vi "Start Triggers Time.vi"(0 "time.resources":T3, 5 "rx.parameters":T9={"rx.trigger select"=enum."Software", "rx.trigger enable"=FALSE, "rx.trigger sync enable"=FALSE, "rx.stream enable"=[FALSE, FALSE, FALSE, FALSE], "rx.software trigger"=FALSE, "rx.reset"=FALSE, "rx.abort"=FALSE, "rx.samples to acquire"=0, "rx.data sink"=enum."SFP Port 0", "rx.ddc parameters"=[{"output sample rate"=0.0, "delay"=0.0, "frequency shift"=0.0, "impairments"={"inline gain I"=0.0, "inline gain Q"=0.0, "cross gain I"=0.0, "cross gain Q"=0.0, "pre-gain offset I"=0.0, "pre-gain offset Q"=0.0, "post-gain offset I"=0.0, "post-gain offset Q"=0.0}, "phase"=0.0}, {"output sample rate"=0.0, "delay"=0.0, "frequency shift"=0.0, "impairments"={"inline gain I"=0.0, "inline gain Q"=0.0, "cross gain I"=0.0, "cross gain Q"=0.0, "pre-gain offset I"=0.0, "pre-gain offset Q"=0.0, "post-gain offset I"=0.0, "post-gain offset Q"=0.0}, "phase"=0.0}, {"output sample rate"=0.0, "delay"=0.0, "frequency shift"=0.0, "impairments"={"inline gain I"=0.0, "inline gain Q"=0.0, "cross gain I"=0.0, "cross gain Q"=0.0, "pre-gain offset I"=0.0, "pre-gain offset Q"=0.0, "post-gain offset I"=0.0, "post-gain offset Q"=0.0}, "phase"=0.0}, {"output sample rate"=0.0, "delay"=0.0, "frequency shift"=0.0, "impairments"={"inline gain I"=0.0, "inline gain Q"=0.0, "cross gain I"=0.0, "cross gain Q"=0.0, "pre-gain offset I"=0.0, "pre-gain offset Q"=0.0, "post-gain offset I"=0.0, "post-gain offset Q"=0.0}, "phase"=0.0}]} {"rx.ddc parameters"."frequency shift" format="%#.48g"}, 7 "tx.parameters":T4={"tx.trigger select"=enum."Software", "tx.trigger enable"=FALSE, "tx.trigger sync enable"=FALSE, "tx.stream enable"=[FALSE, FALSE], "tx.software trigger"=FALSE, "tx.reset"=FALSE, "tx.abort"=FALSE, "tx.samples to generate"=0, "tx.data source"=enum."SFP Port 0", "tx.duc parameters"=[{"frequency shift"=0.0, "impairments"={"inline gain I"=0.0, "inline gain Q"=0.0, "cross gain I"=0.0, "cross gain Q"=0.0, "pre-gain offset I"=0.0, "pre-gain offset Q"=0.0, "post-gain offset I"=0.0, "post-gain offset Q"=0.0}, "phase"=0.0, "input sample rate"=0.0, "gain"={"gain I"=0.0, "gain Q"=0.0}, "delay"=0.0}, {"frequency shift"=0.0, "impairments"={"inline gain I"=0.0, "inline gain Q"=0.0, "cross gain I"=0.0, "cross gain Q"=0.0, "pre-gain offset I"=0.0, "pre-gain offset Q"=0.0, "post-gain offset I"=0.0, "post-gain offset Q"=0.0}, "phase"=0.0, "input sample rate"=0.0, "gain"={"gain I"=0.0, "gain Q"=0.0}, "delay"=0.0}]} {"tx.duc parameters"."frequency shift" format="%#.48g"}) -> (4 "rx.start trigger":bool, 6 "tx.start trigger":bool)   [LabVIEW 2018]
doc: "Generates start triggers for Rx and Tx. Start triggers are generated based on which trigger type is selected, whether the stream is enabled, whether triggers are enabled, and whether the triggers are to be synchronized across multiple devices.\n\n<B>Input Parameters</B>\n\n<B>enable stream</B> controls the output of a 'start trigger'.\n\n<B>software trigger</B> is a start trigger asserted by software.\n\n<B>enable trigger</B> controls the output of a 'start trigger'.\n\n<B>enable trigger sync</B> to synchronize a 'start trigger' between multiple devices. The master device sends the 'start trigger' to all the slave devices. If enabled, the slave devices ignore the 'trigger select' because the 'start trigger' from the master device is used instead.\n\n<B>trigger select</B> picks which source to use as the 'start trigger'.\n\n<B>Output Parameters</B>\n\n<B>rx.start trigger</B> is the signal to use at the 'start trigger' for the Rx data path.\n\n<B>tx.start trigger</B> is the signal to use at the 'start trigger' for the Tx data path."
uses:
  Rx Parameters.ctl
  Host/SubVIs/Start Trigger.ctl
  DDC Parameters.ctl
  <instrlib>/_niInstr/DSP/v1/Shared/Public/IQ Impairments.ctl
  Tx Parameters.ctl
  DUC Parameters.ctl
  <instrlib>/_niInstr/DSP/v1/Shared/Public/IQ Gain.ctl
  <instrlib>/niUsrpRio/Time/v1/FPGA/Private/Time Resources.ctl
  <instrlib>/niUsrpRio/Time/v1/FPGA/Private/Future Event Resources.ctl
  <instrlib>/_niInstr/DSP/v1/Shared/niInstr DSP v1 Shared.lvlib
  <instrlib>/niUsrpRio/Time/v1/FPGA/niUsrpRio Time v1 FPGA.lvlib
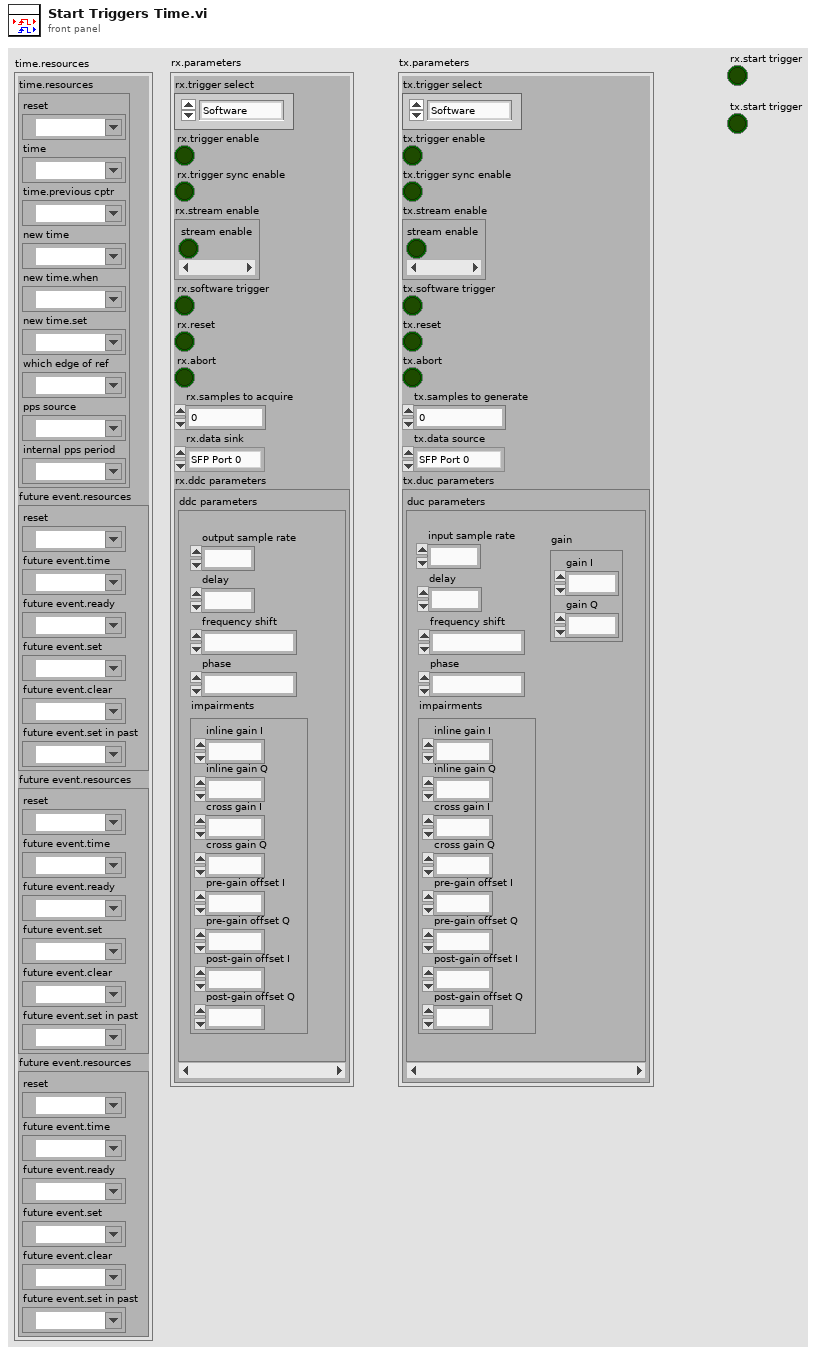
[diagram p1: front panel]
types:
  T1 = typedef "niUsrpRio Time v1 FPGA.lvlib/Time Resources.ctl" = cluster{"reset":refnum<k21>, "time":refnum<k21>, "time.previous cptr":refnum<k21>, "new time":refnum<k21>, "new time.when":refnum<k21>, "new time.set":refnum<k21>, "which edge of ref":refnum<k21>, "pps source":refnum<k21>, "internal pps period":refnum<k21>}
  T2 = typedef "niUsrpRio Time v1 FPGA.lvlib/Future Event Resources.ctl" = cluster{"reset":refnum<k21>, "future event.time":refnum<k21>, "future event.ready":refnum<k21>, "future event.set":refnum<k21>, "future event.clear":refnum<k21>, "future event.set in past":refnum<k21>}
  T3 = cluster{"time.resources":T1, "future event.resources":T2, "future event.resources":T2, "future event.resources":T2}
  T4 = typedef "Tx Parameters.ctl" = cluster{"tx.trigger select":T5, "tx.trigger enable":bool, "tx.trigger sync enable":bool, "tx.stream enable":bool[], "tx.software trigger":bool, "tx.reset":bool, "tx.abort":bool, "tx.samples to generate":u32, "tx.data source":enum16{"SFP Port 0", "SFP Port 1", "Host"}, "tx.duc parameters":T6[]}
  T5 = typedef "Start Trigger.ctl" = enum8{"Software", "Digital Edge", "Rx Start Trigger", "Tx Start Trigger", "Immediate", "Future Time Event"}
  T6 = typedef "DUC Parameters.ctl" = cluster{"frequency shift":fxp<+/-,48,0>, "impairments":T7, "phase":fxp<+/-,21,0>, "input sample rate":fxp<+,48,1>, "gain":T8, "delay":fxp<+/-,18,0>}
  T7 = typedef "niInstr DSP v1 Shared.lvlib/IQ Impairments.ctl" = cluster{"inline gain I":fxp<+/-,18,1>, "inline gain Q":fxp<+/-,18,1>, "cross gain I":fxp<+/-,18,1>, "cross gain Q":fxp<+/-,18,1>, "pre-gain offset I":fxp<+/-,18,1>, "pre-gain offset Q":fxp<+/-,18,1>, "post-gain offset I":fxp<+/-,18,1>, "post-gain offset Q":fxp<+/-,18,1>}
  T8 = typedef "niInstr DSP v1 Shared.lvlib/IQ Gain.ctl" = cluster{"gain I":fxp<+/-,24,3>, "gain Q":fxp<+/-,24,3>}
  T9 = typedef "Rx Parameters.ctl" = cluster{"rx.trigger select":T5, "rx.trigger enable":bool, "rx.trigger sync enable":bool, "rx.stream enable":bool[], "rx.software trigger":bool, "rx.reset":bool, "rx.abort":bool, "rx.samples to acquire":u32, "rx.data sink":enum16{"SFP Port 0", "SFP Port 1", "Host"}, "rx.ddc parameters":T10[]}
  T10 = typedef "DDC Parameters.ctl" = cluster{"output sample rate":fxp<+,48,1>, "delay":fxp<+/-,16,0>, "frequency shift":fxp<+/-,48,0>, "impairments":T7, "phase":fxp<+/-,21,0>}
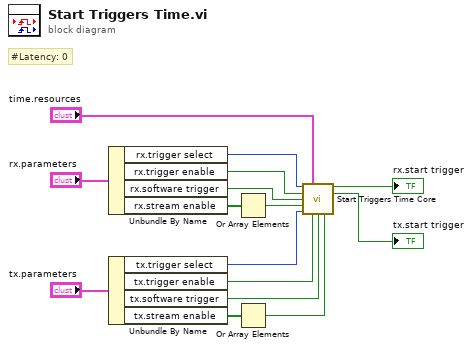
[diagram p0: block diagram]
diagram:
  # "#Latency: 0"
  n1 = Unbundle By Name("rx.parameters") -> ("rx.trigger select"=w11:T5, "rx.trigger enable"=w10:bool, "rx.software trigger"=w9:bool, "rx.stream enable"=w8:bool[])
  n2 = Unbundle By Name("tx.parameters") -> ("tx.trigger select"=w6:T5, "tx.trigger enable"=w5:bool, "tx.software trigger"=w4:bool, "tx.stream enable"=w3:bool[])
  n3 = Or Array Elements(Boolean array=w8) -> (logical OR=w7:bool)
  n4 = Or Array Elements(Boolean array=w3) -> (logical OR=w2:bool)
  n5 = call "Start Triggers Time Core.vi"("rx.trigger select"=w11, "time.resources"="time.resources", "rx.trigger enable"=w10, "rx.software trigger"=w9, "rx.stream enable"=w7, "tx.trigger select"=w6, "tx.trigger enable"=w5, "tx.software trigger"=w4, "tx.stream enable"=w2) -> ("rx.start trigger"=→"rx.start trigger":bool, "tx.start trigger"=→"tx.start trigger":bool)  [unwired: 5 in]
